vi "Reformat.vi"(4 "Disable LabVIEW Extensions":bool, 5 "Format empty string as null":bool, 6 "Pretty Print Levels":i32, 7 "Alphabetically Sort Objects":bool, 8 "error in (no error)":errorcluster, 10 "Offset":i32, 11 "JSON":string) -> (0 "error out":errorcluster, 1 "Offset past":i32 caption="Offset past Value", 2 "Rest of Input String":string, 3 "<JSON>":string caption="<JSON>First JSON Value")   [LabVIEW 2021, in "json.facade.lvlib"]
doc: "Reformat a JSON Value, either packed with all unneeded whitespace removed, or \"pretty printed\" with extra whitespace and new lines to make the JSON more human readable. This will also serve to validate the JSON.\n\n\"Pretty Print Levels\" is the number of deeper levels at which to apply pretty print. Use a high number to apply at all levels, and use zero to indicate no pretty print."
uses:
  json.facade.lvlib
  jsontext/JSONtext.lvlib
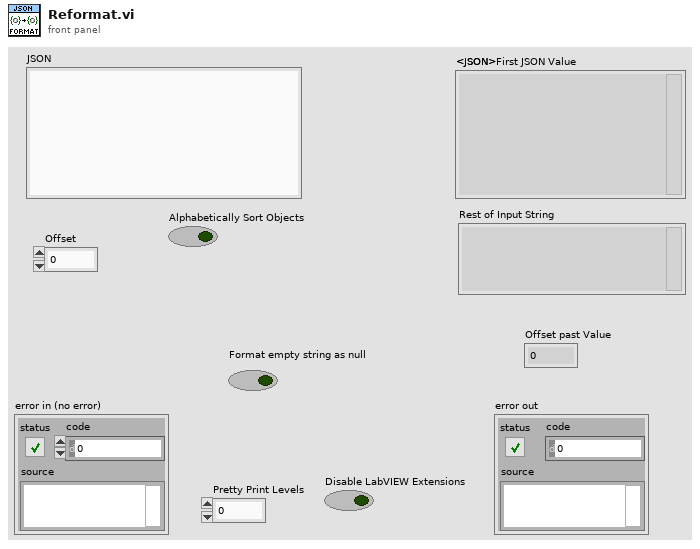
[diagram p1: front panel]
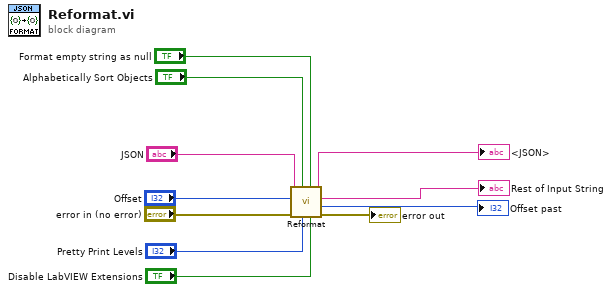
[diagram p0: block diagram]
diagram:
  n1 = call "Reformat.vi"("Disable LabVIEW Extensions"="Disable LabVIEW Extensions", "Format empty string as null"="Format empty string as null", "Pretty Print Levels"="Pretty Print Levels", "Alphabetically Sort Objects"="Alphabetically Sort Objects", "error in (no error)"="error in (no error)", "Offset"="Offset", "JSON"="JSON") -> ("error out"=→"error out":errorcluster, "Offset past"=→"Offset past":i32, "Rest of Input String"=→"Rest of Input String":string, "<JSON>"=→"<JSON>":string)  [unwired: 1 in]
